vi "COMI SD502 Clear Multi.vi"(10 "dwCtrlBits":u32, 11 "hDevice":u32) -> (3 "hDevice out":u32)   [LabVIEW 2017, in "Comidll.lvlib"]
doc: "void (COMI_SD502_ClearMulti) (HANDLE hDevice, unsigned long dwCtrlBits);"
uses:
  <userlib>/Comidll/Comidll.lvlib
  <userlib>/Comidll/Comidll.dll
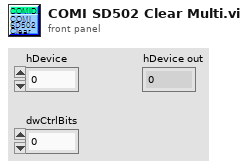
[diagram p1: front panel]
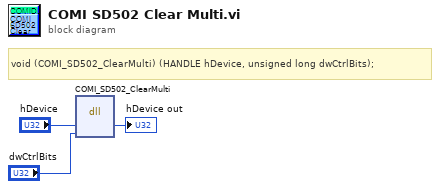
[diagram p0: block diagram]
diagram:
  # "void\t(COMI_SD502_ClearMulti) (HANDLE hDevice, unsigned long dwCtrlBits);"
  n1 = dll-call lib="C:/Program Files/National Instruments/LabVIEW 2017/user.lib/Comidll/Comidll.*" fn="COMI_SD502_ClearMulti"("hDevice"="hDevice", "dwCtrlBits"="dwCtrlBits") -> ("hDevice"=→"hDevice out":u32)  [unwired: 5 in, 2 out]
